vi "Motor Control Message Loop.vi"(8 "error in (no error)":errorcluster caption="错误输入（无错误）", 11 "Message Queues":T1 caption="消息队列") -> (0 "error out":errorcluster caption="错误输出")   [LabVIEW 2015, in "Motor Control.lvlib"]
doc: "该消息循环负责处理硬件数据采集的相关消息。"
uses:
  Motor Control.lvlib
  support/Message Queue/All Message Queues.ctl
  support/Message Queue/Message Cluster.ctl
  Hardware Configuration.ctl
  Motor Control State.ctl
  support/Message Queue/Enqueue Message (Single).vi
  <vilib>/Utility/error.llb/Error Cluster From Error Code.vi
  <vilib>/ErrorRing/Error Ring.xnode
  support/Message Queue/Message Queue.lvlib
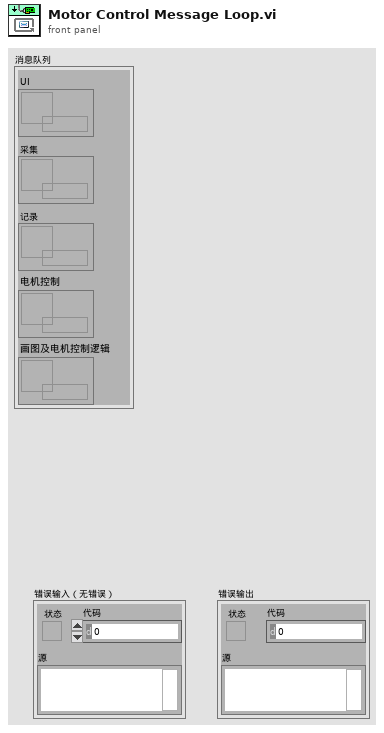
[diagram p1: front panel]
types:
  T1 = typedef "Message Queue.lvlib/All Message Queues.ctl" = cluster{"UI":refnum<queue>, "Acquisition":refnum<queue>, "Logging":refnum<queue>, "MotorCtrl":refnum<queue>, "plot logic":refnum<queue>}
  T2 = typedef "Motor Control.lvlib/Hardware Configuration.ctl" = cluster{"counter":tag, "方向端口":tag, "当前方向":bool, "频率":dbl, "DAQmx Task":refnum<k21>}
  T3 = typedef "Motor Control.lvlib/Motor Control State.ctl" = enum16{"Idle", "Acquiring"}
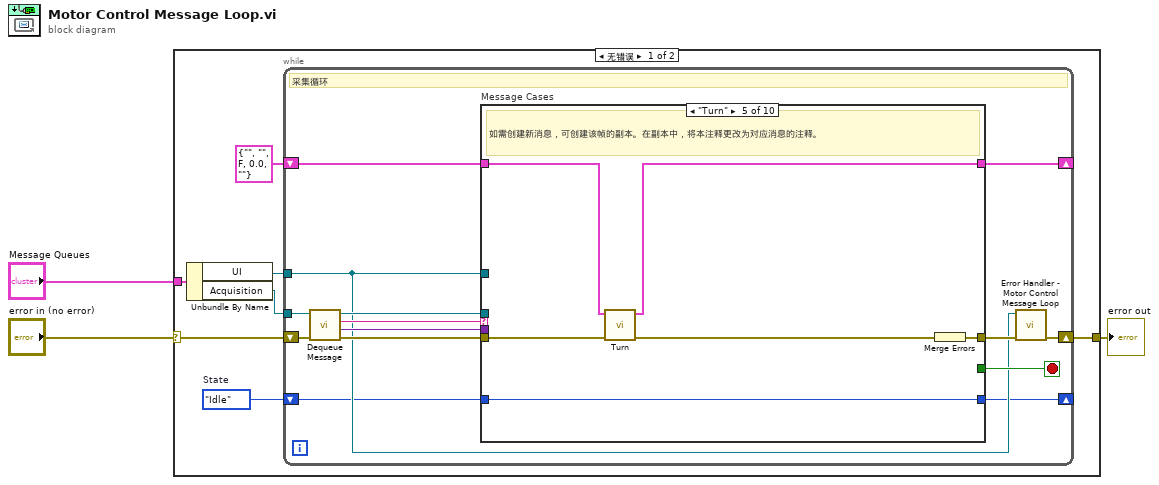
[diagram p0: block diagram]
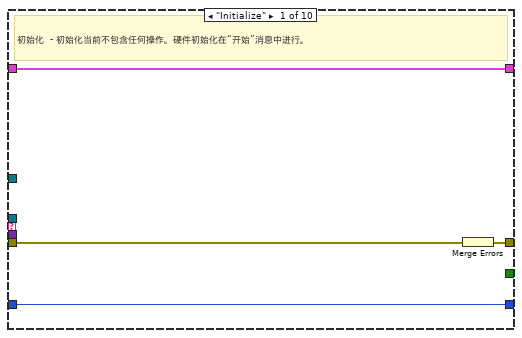
[diagram p2: hidden frame]
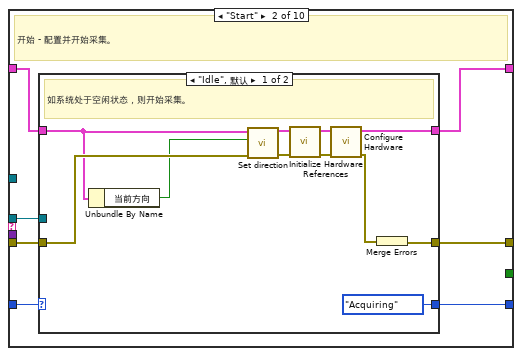
[diagram p3: hidden frame]
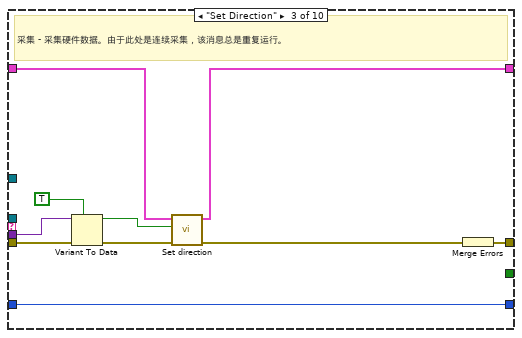
[diagram p5: hidden frame]
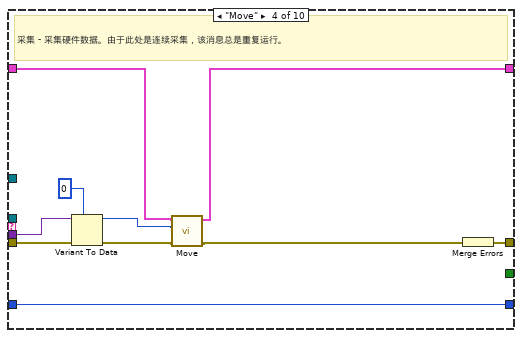
[diagram p6: hidden frame]
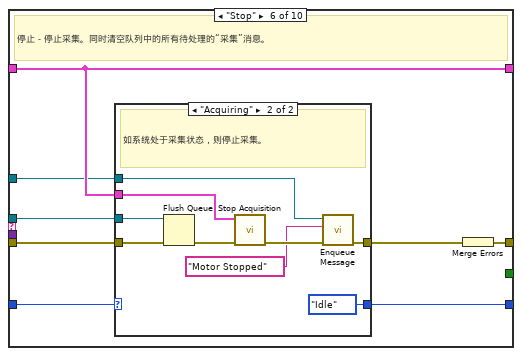
[diagram p7: hidden frame]
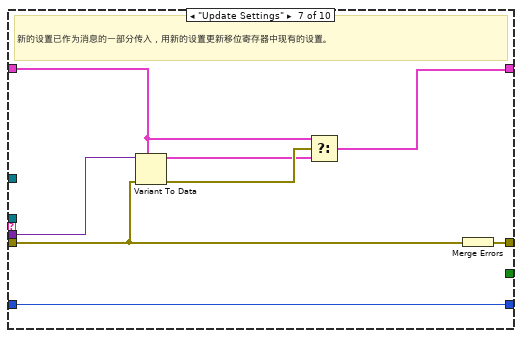
[diagram p9: hidden frame]
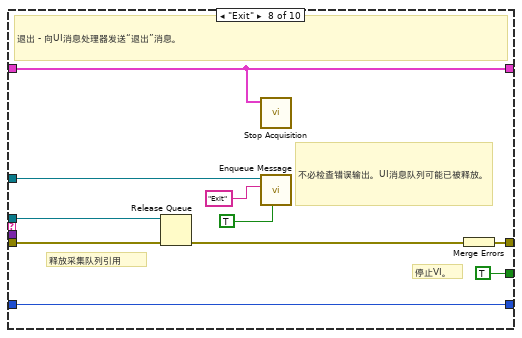
[diagram p10: hidden frame]
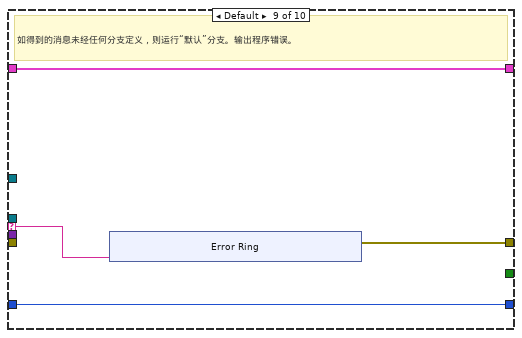
[diagram p11: hidden frame]
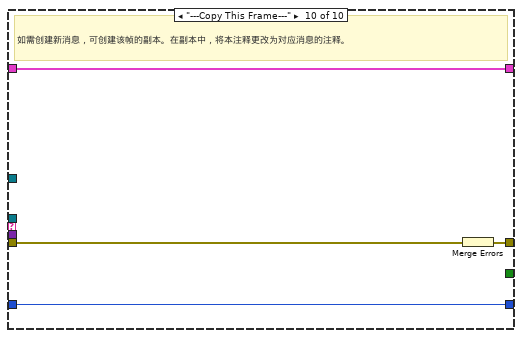
[diagram p12: hidden frame]
diagram:
  n1 = case shown="无错误" "error in (no error)" {
    selector: "error in (no error)" -> [w6 w128]
    tunnel: "Message Queues" -> [w10 _]
    tunnel: [w8 w128] -> w2
    frame No Error {
      w4 = Motor_Control_State."Idle"  # State
      n2 = Unbundle By Name(w10) -> ("UI"=w5:refnum<queue>, "Acquisition"=w9:refnum<queue>)
      n3 = while {
        tunnel: w9 -> [w16]
        shift-right: [w23] -> _
        shift-left: T2 {"counter"="", "方向端口"="", "当前方向"=FALSE, "频率"=0.0, "DAQmx Task"=""} ("Data Cluster") -> [w24]
        shift-right: [w14] -> w8
        shift-left: w6 -> [w21]
        tunnel: w5 -> [w13]
        shift-right: [w11] -> _
        shift-left: w4 -> [w12]
        stop <- w22 stop-if-true
        # "采集循环"
        n4 = call "Dequeue Message.vi"("error in (no error)"=w21, "Message Queue"=w16) -> ("error out"=w20:errorcluster, "Message Data"=w18:variant, "Message"=w19:string, "dup Message Queue"=w17:refnum<queue>)  [unwired: 6 in]
        n5 = case "Message Cases" shown="\"Turn\"" w19 {
          selector: w19 -> [_ _ _ _ _ _ _ _ w115 _]
          tunnel: w17 -> [_ w32 _ _ _ w80 _ w105 _ _]
          tunnel: w20 -> [w27 w33 w57 w67 w73 w82 w96 w109 _ w127]
          tunnel: [w28 w35 w59 w69 w75 w83 w102 w111 w114 w125] -> w15
          tunnel: w24 -> [w26 w34 w52 w65 w71 w81 w98 w104 w116 w126]
          tunnel: [w26 w31 w50 w64 w70 w81 w97 w104 w116 w126] -> w23
          tunnel: [_ _ _ _ _ _ _ TRUE _ _] -> w22
          tunnel: w18 -> [_ _ w56 w66 _ _ w101 _ _ _]
          tunnel: w13 -> [_ _ _ _ _ w79 _ w110 _ _]
          tunnel: w12 -> [w25 w30 w58 w68 w74 w78 w95 w103 w113 w124]
          tunnel: [w25 w29 w58 w68 w74 w77 w95 w103 w113 w124] -> w11
          frame "Initialize" {
            # "初始化  - 初始化当前不包含任何操作。硬件初始化在“开始”消息中进行。"
            n6 = Merge Errors(w27) -> (w28:errorcluster)
          }
          frame "Start" {
            # "开始 - 配置并开始采集。"
            n7 = case shown="\"Idle\", 默认" w30 {
              selector: w30 -> [_ w47]
              tunnel: [w46 w49] -> w35
              tunnel: w34 -> [w37 w48]
              tunnel: w33 -> [w38 w49]
              tunnel: w32 -> [_ _]
              tunnel: [w42 w48] -> w31
              tunnel: [Motor_Control_State."Acquiring" ("State") w47] -> w29
              frame "Idle", Default {
                # "如系统处于空闲状态，则开始采集。"
                n8 = Unbundle By Name(w37) -> ("当前方向"=w36:bool)
                n9 = call "Set direction.vi"("error in (no error)"=w38, "方向"=w36, "Hardware Resources in"=w37) -> ("error out"=w39:errorcluster, "Hardware Resources out"=w40:T2)  [unwired: 7 in]
                n10 = call "Initialize Hardware References.vi"("error in (no error)"=w39, "Hardware Resources in"=w40) -> ("error out"=w45:errorcluster, "Hardware Resources out"=w43:T2)  [unwired: 8 in]
                n11 = call "Configure Hardware.vi"("error in (no error)"=w45, "Hardware Resources in"=w43) -> ("error out"=w44:errorcluster, "Hardware Resources out"=w42:T2)  [unwired: 8 in]
                n12 = Merge Errors(w44) -> (w46:errorcluster)
              }
              frame "Acquiring" {
                # "系统已开始采集。忽略“开始”消息。"
              }
            }
          }
          frame "Set Direction" {
            # "采集 - 采集硬件数据。由于此处是连续采集，该消息总是重复运行。"
            n13 = Variant To Data(error in=w57, type=TRUE, Variant=w56) -> (data=w51:bool, error out=w54:errorcluster)
            n14 = call "Set direction.vi"("error in (no error)"=w54, "方向"=w51, "Hardware Resources in"=w52) -> ("error out"=w53:errorcluster, "Hardware Resources out"=w50:T2)  [unwired: 7 in]
            n15 = Merge Errors(w53) -> (w59:errorcluster)
          }
          frame "Move" {
            # "采集 - 采集硬件数据。由于此处是连续采集，该消息总是重复运行。"
            n16 = Variant To Data(error in=w67, type=0, Variant=w66) -> (data=w63:i32, error out=w62:errorcluster)
            n17 = call "Move.vi"("error in (no error)"=w62, "samples per channel"=w63, "Hardware Resources in"=w65) -> ("error out"=w61:errorcluster, "Hardware Resources out"=w64:T2)  [unwired: 7 in]
            n18 = Merge Errors(w61) -> (w69:errorcluster)
          }
          frame "Turn" {
            # "如需创建新消息，可创建该帧的副本。在副本中，将本注释更改为对应消息的注释。"
            n19 = call "Turn.vi"("error in (no error)"=w73, "Hardware Resources in"=w71) -> ("error out"=w72:errorcluster, "Hardware Resources out"=w70:T2)  [unwired: 8 in]
            n20 = Merge Errors(w72) -> (w75:errorcluster)
          }
          frame "Stop" {
            # "停止－停止采集。同时清空队列中的所有待处理的“采集”消息。"
            n21 = case shown="\"Acquiring\"" w78 {
              selector: w78 -> [w85 _]
              tunnel: w82 -> [w84 w94]
              tunnel: w81 -> [_ w93]
              tunnel: w80 -> [_ w91]
              tunnel: w79 -> [_ w90]
              tunnel: [w85 Motor_Control_State."Idle" ("State")] -> w77
              tunnel: [w84 w88] -> w76
              frame "Idle", Default {
                # "系统已处于空闲状态。忽略“停止”消息。"
              }
              frame "Acquiring" {
                # "如系统处于采集状态，则停止采集。"
                n22 = Flush Queue(queue=w91, error in (no error)=w94) -> (error out=w92:errorcluster)  [unwired: 2 out]
                n23 = call "Stop Acquisition.vi"("error in (no error)"=w92, "Hardware Resources in"=w93) -> ("error out"=w89:errorcluster)  [unwired: 9 in]
                n24 = call-poly "Enqueue Message.vi"("error in (no error)"=w89, "Message"="Motor Stopped", "Message Queue"=w90) -> ("error out"=w88:errorcluster)  [unwired: 7 in, 1 out]
              }
            }
            n25 = Merge Errors(w76) -> (w83:errorcluster)
          }
          frame "Update Settings" {
            # "新的设置已作为消息的一部分传入，用新的设置更新移位寄存器中现有的设置。"
            n26 = Variant To Data(error in=w96, type=w98, Variant=w101) -> (data=w99:T2, error out=w100:errorcluster)
            n27 = Select(t=w98, s=w100, f=w99) -> (s? t:f=w97:T2)
            n28 = Merge Errors(w96) -> (w102:errorcluster)
          }
          frame "Exit" {
            # "不必检查错误输出。UI消息队列可能已被释放。"
            # "释放采集队列引用"
            # "停止VI。"
            # "退出 - 向UI消息处理器发送“退出”消息。"
            n29 = Release Queue(queue=w105, error in (no error)=w109) -> (error out=w106:errorcluster)  [unwired: 1 in, 2 out]
            n30 = call "Stop Acquisition.vi"("Hardware Resources in"=w104) -> ()  [unwired: 10 in, 1 out]
            n31 = call-poly "Enqueue Message.vi"("Priority Message? (F)"=TRUE, "Message"="Exit", "Message Queue"=w110) -> ()  [unwired: 7 in, 2 out]
            n32 = Merge Errors(w106) -> (w111:errorcluster)
          }
          frame Default {
            # "如得到的消息未经任何分支定义，则运行“默认”分支。输出程序错误。"
            n33 = xnode "Error Ring"("参数 0"=w115) -> ("错误输出"=w114:errorcluster)
          }
          frame "---Copy This Frame---" {
            # "如需创建新消息，可创建该帧的副本。在副本中，将本注释更改为对应消息的注释。"
            n34 = Merge Errors(w127) -> (w125:errorcluster)
          }
        }
        n35 = call "Error Handler - Motor Control Message Loop.vi"("error in (no error)"=w15, "Message Queue"=w13) -> ("dup error in"=w14:errorcluster)  [unwired: 8 in, 1 out]
      }
    }
    frame Error {
    }
  }
  "error out" <- w2
